vi "Read_Electrical_Variables_v2[Conflict].vi"(8 "error in (no error)":errorcluster, 11 "Modbus master in":refnum<class "Modbus Master.lvclass">) -> (0 "error out":errorcluster, 2 "Variables":sgl[](array[numeric]), 3 "Modbus master out":refnum<class "Modbus Master.lvclass">)   [LabVIEW 2018]
uses:
  <vilib>/Modbus/master/Modbus Master.lvclass
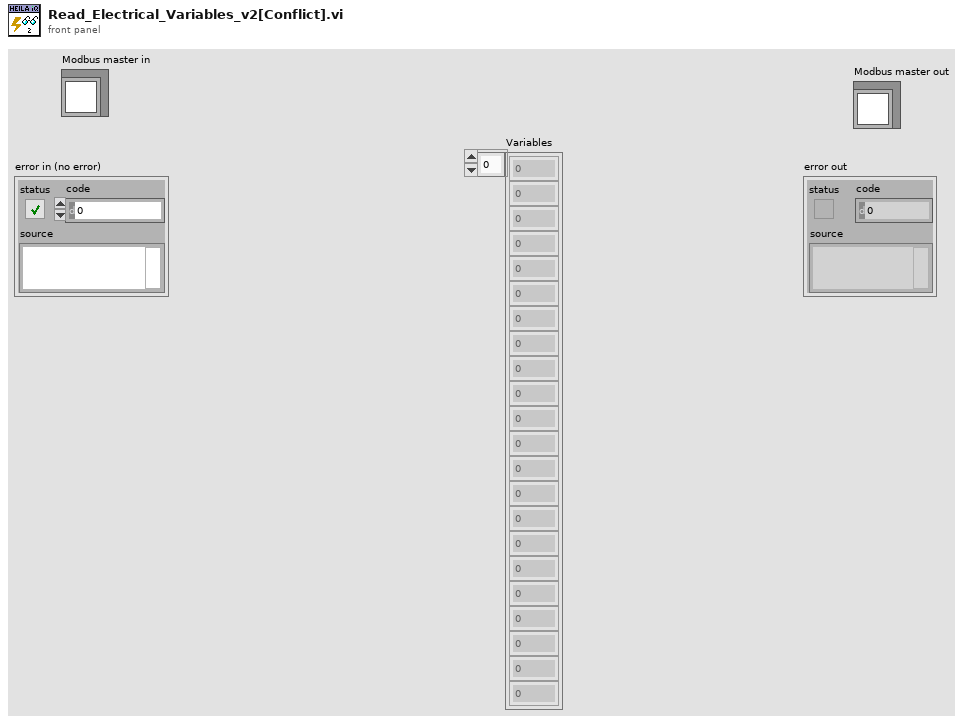
[diagram p1: front panel]
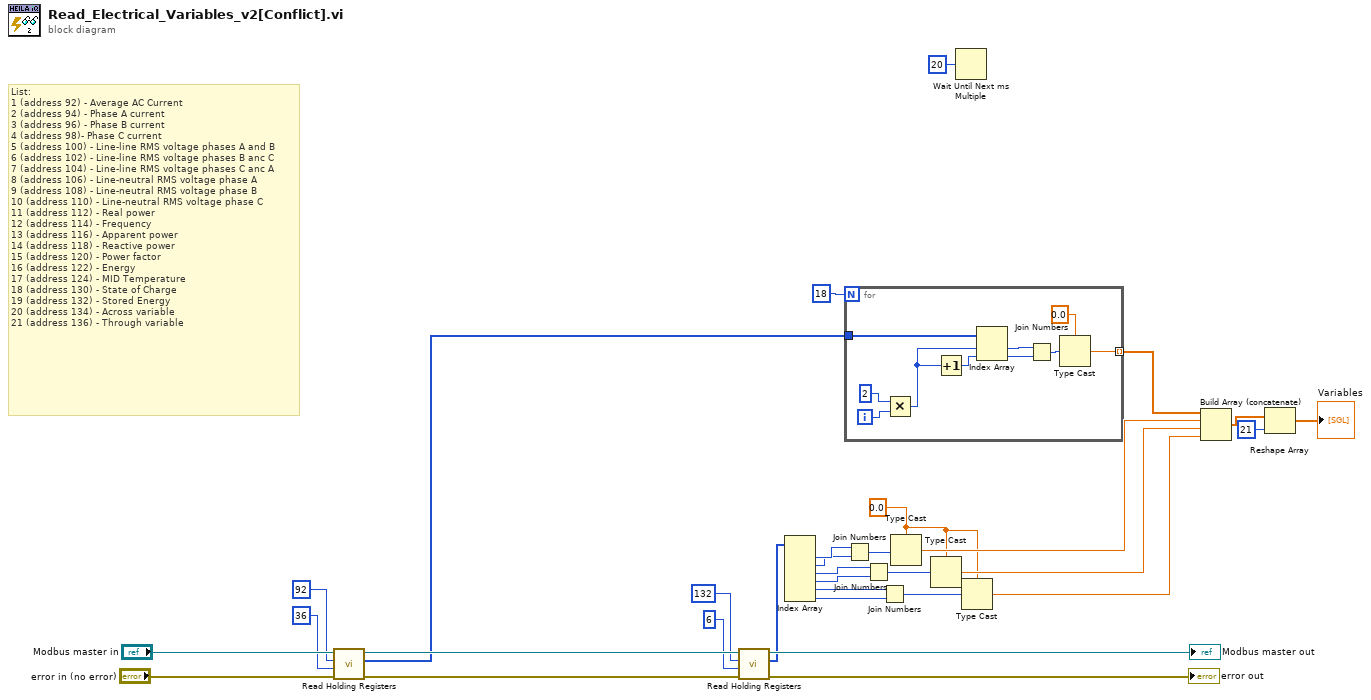
[diagram p0: block diagram]
diagram:
  w2 = sgl 0.0
  # "List:\n1 (address 92) - Average AC Current\n2 (address 94) - Phase A current\n3 (address 96) - Phase B current\n4 (address 98)- Phase C current\n5 (address 100) - Line-line RMS voltage phases A and B\n6 (address 102) - Line-line RMS voltage phases B anc C\n7 (address 104) - Line-line RMS voltage phases C anc A\n8 (address 106) - Line-neutral RMS voltage phase A\n9 (address 108) - Line-neutral RMS voltage phase B\n10 (address 110) - Line-neutral RMS voltage phase C\n11 (address 112) - Real power\n12 (address 114) - Frequency\n13 (address 116) - Apparent power\n14 (address 118) - Reactive power\n15 (address 120) - Power factor\n16 (address 122) - Energy\n17 (address 124) - MID Temperature\n18 (address 130) - State of Charge\n19 (address 132) - Stored Energy\n20 (address 134) - Across variable\n21 (address 136) - Through variable"
  n1 = call-dynamic "Read Holding Registers.vi"("error in (no error)"="error in (no error)", "number of holding registers"=u16 36 ("starting address"), "starting address"=u16 92, "Modbus master in"="Modbus master in") -> ("error out"=w26:errorcluster, "register values"=w16:u16[], "Modbus master out"=w27:refnum<class "Modbus Master.lvclass">)  [unwired: 5 in]
  n2 = call-dynamic "Read Holding Registers.vi"("error in (no error)"=w26, "number of holding registers"=u16 6 ("starting address"), "starting address"=u16 132, "Modbus master in"=w27) -> ("error out"=→"error out":errorcluster, "register values"=w21:u16[], "Modbus master out"=→"Modbus master out":refnum<class "Modbus Master.lvclass">)  [unwired: 5 in]
  n3 = Index Array(array=w21) -> (element #1=w20:u16, element #2=w19:u16, element #3=w10:u16, element #4=w9:u16, element #5=w8:u16, element #6=w7:u16)  [unwired: 6 in]
  n4 = for {
    N: 18 -> [_]
    tunnel: [w37] -> w15 mode=indexing
    tunnel: w16 -> [w32]
    i -> [w36]
    n5 = Multiply(x=2, y=w36) -> (x*y=w33:i32)
    n6 = Increment(x=w33) -> (x+1=w34:i32)
    n7 = Index Array(array=w32, index #1=w33, index #2=w34) -> (element #1=w41:u16, element #2=w40:u16)
    n8 = Join Numbers(hi=w41, lo=w40) -> ((hi.lo)=w38:u32)
    n9 = Type Cast(type=sgl 0.0, x=w38) -> (*(type *) &x=w37:sgl)
  }
  n10 = Join Numbers(hi=w20, lo=w19) -> ((hi.lo)=w18:u32)
  n11 = Join Numbers(hi=w10, lo=w9) -> ((hi.lo)=w6:u32)
  n12 = Join Numbers(hi=w8, lo=w7) -> ((hi.lo)=w5:u32)
  n13 = Type Cast(type=w2, x=w18) -> (*(type *) &x=w14:sgl)
  n14 = Type Cast(type=w2, x=w6) -> (*(type *) &x=w4:sgl)
  n15 = Wait Until Next ms Multiple(millisecond multiple=u32 20) -> ()  [unwired: 1 out]
  n16 = Type Cast(type=w2, x=w5) -> (*(type *) &x=w3:sgl)
  n17 = Build Array (concatenate)(w15, w14, w4, w3) -> (w13:sgl[])
  n18 = Reshape Array(w13, 21 ("dimension size")) -> (→"Variables":sgl[])
